vi "Restart.LoadSettings.vi"(8 "error in":errorcluster, 11 "path (use dialog)":path) -> (0 "error out":errorcluster, 2 "Restart Settings":T1={"LogFile"=path "", "Log Settings"=[], "StimulusProfile"=path "", "StopIteration"=0, "StopStep"=0, "Log Channels"=enum."Aliases", "Base File Name"="Log", "Enable Logging"=TRUE, "Profile"="", "StopDuration"=0.0}, 3 "path":path)   [LabVIEW 2013, in "Simple Sequence Tools - Execution.lvlib"]
uses:
  Simple Sequence Tools - Execution.lvlib
  Types/Restart.Settings
  <vilib>/NI Veristand/Execution/DataLogging/TDMS Channel Group.ctl
  <vilib>/NI Veristand/Execution/DataLogging/TDMS Property.ctl
  <vilib>/NI Veristand/Execution/DataLogging/TDMS Channel.ctl
  <vilib>/NI Veristand/Execution/DataLogging/Time Channel Options.ctl
  Types/Log.SelectedChannels.ctl
  Shared/SubVIs/Main.Constants.vi
  <vilib>/NI/GXML/_subVIs/GXML Quick Parser/Quick Parser.vi
  <vilib>/NI/GXML/GXML.lvlib
  Shared/Simple Sequence Tools - Shared.lvlib
  <vilib>/NI Veristand/Execution/DataLogging/NI_VS Data Logging API.lvlib
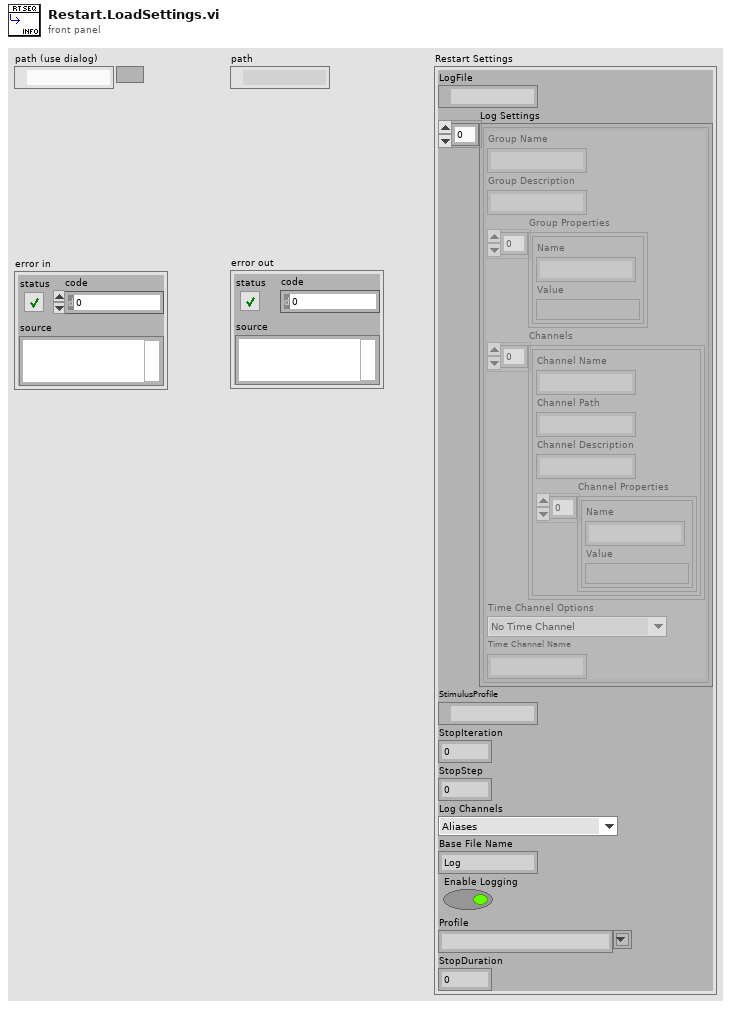
[diagram p1: front panel]
types:
  T1 = typedef "Simple Sequence Tools - Execution.lvlib/Restart.Settings" = cluster{"LogFile":path, "Log Settings":T2[], "StimulusProfile":path, "StopIteration":u32, "StopStep":u32, "Log Channels":T6, "Base File Name":string, "Enable Logging":bool, "Profile":string, "StopDuration":dbl}
  T2 = typedef "NI_VS Data Logging API.lvlib/TDMS Channel Group.ctl" = cluster{"Group Name":string, "Group Description":string, "Group Properties":T3[], "Channels":T4[], "Time Channel Options":T5, "Time Channel Name":string}
  T3 = typedef "NI_VS Data Logging API.lvlib/TDMS Property.ctl" = cluster{"Name":string, "Value":variant}
  T4 = typedef "NI_VS Data Logging API.lvlib/TDMS Channel.ctl" = cluster{"Channel Name":string, "Channel Path":string, "Channel Description":string, "Channel Properties":T3[]}
  T5 = typedef "NI_VS Data Logging API.lvlib/Time Channel Options.ctl" = enum16{"No Time Channel", "Absolute Time", "System Time", "System Time - Microseconds", "Absolute Time as Double"}
  T6 = typedef "Simple Sequence Tools - Execution.lvlib/Log.SelectedChannels.ctl" = enum16{"Channels (No System Channel)", "Aliases", "All"}
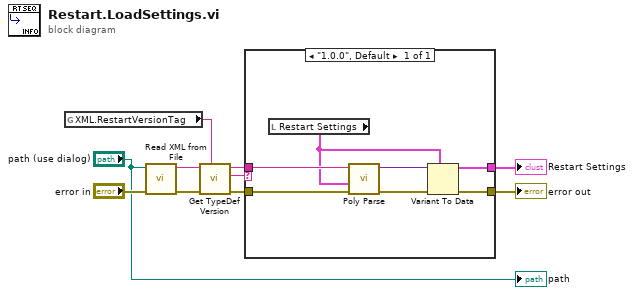
[diagram p0: block diagram]
diagram:
  n1 = global read "Main.Constants.vi" "XML.RestartVersionTag"() -> (w5:string)
  n2 = call <vilib>:"Read XML from File.vi"("error in"="error in", "XML File Path"="path (use dialog)") -> ("error out"=w10:errorcluster, "XML String Out"=w8:string)  [unwired: 8 in]
  n3 = call <vilib>:"Get TypeDef Version.vi"("Version Tag Name"=w5, "error in"=w10, "XML String In"=w8) -> ("error out"=w9:errorcluster, "Version String"=w6:string, "XML String Out"=w7:string)  [unwired: 6 in]
  n4 = case shown="\"1.0.0\", Default" w6 {
    tunnel: w9 -> [w15]
    tunnel: w7 -> [w14]
    tunnel: [w13] -> w4
    tunnel: [w12] -> w3
    frame "1.0.0", Default {
      n5 = local read "Restart Settings"() -> (w11:T1)
      n6 = call-poly <vilib>:"Poly Parse.vi"("error in"=w15, "TypeDesc"=w11, "XML File String"=w14) -> ("error out"=w17:errorcluster, "Parsed Data"=w16:variant)  [unwired: 7 in]
      n7 = Variant To Data(error in=w17, type=w11, Variant=w16) -> (data=w13:T1, error out=w12:errorcluster)
    }
  }
  "Restart Settings" <- w4
  "error out" <- w3
  "path" <- "path (use dialog)"
